vi "Manage logger file txt.vi"(0 "length":i32=1 min=1, 5 "Message to add":string, 11 "error in":errorcluster) -> (15 "error out":errorcluster)   [LabVIEW 2020]
panel:
  out "String":string
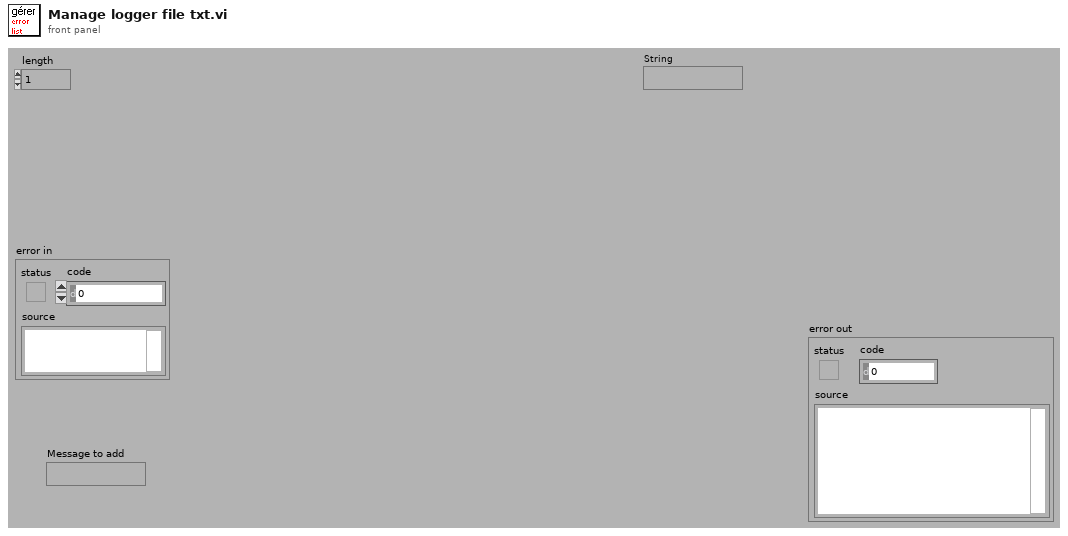
[diagram p1: front panel]
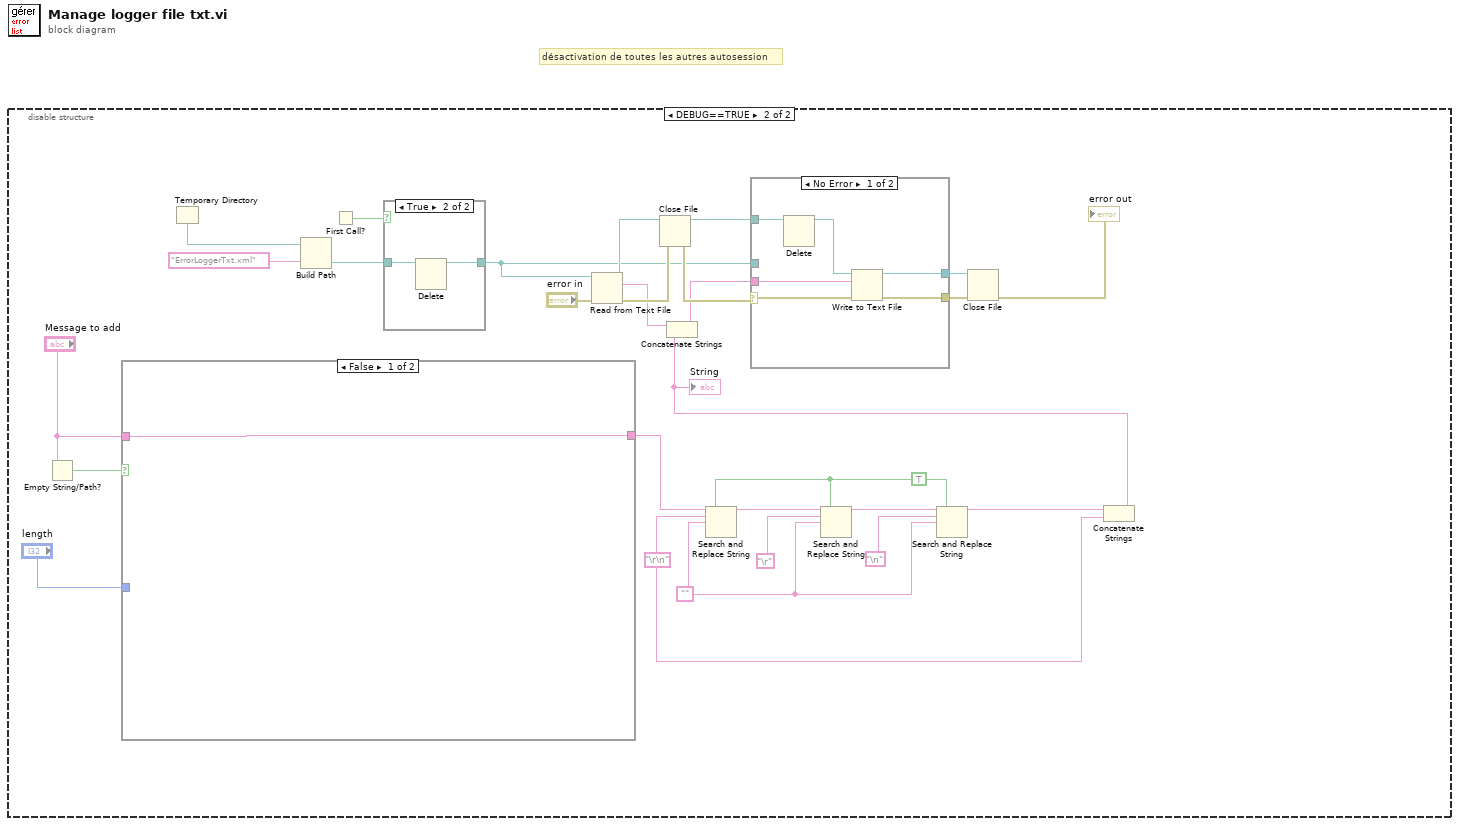
[diagram p0: block diagram]
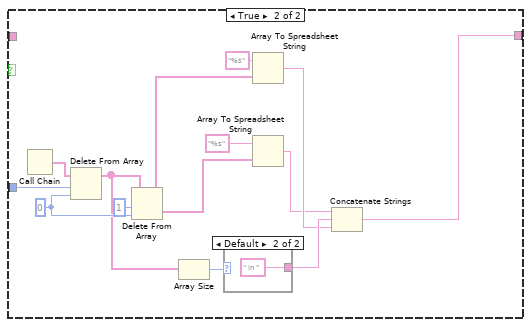
[diagram p3: hidden frame]
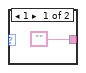
[diagram p4: hidden frame]
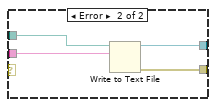
[diagram p6: hidden frame]
diagram:
  # "désactivation de toutes les autres autosession"
  n1 = disable-structure shown="DEBUG==TRUE" {
    frame condition #0 (active) {
    }
    frame condition #1 {
      w2 = "\r\n"
      w4 = ""
      w6 = TRUE ("replace all? (F)")
      n2 = Empty String/Path?(string/path="Message to add") -> (empty?=w13:bool)
      n3 = case shown="False" w13 {
        tunnel: [w29 w35] -> w1
        tunnel: "Message to add" -> [w29 _]
        tunnel: "length" -> [_ w34]
        frame False {
        }
        frame True {
          w39 = 0 ("Index")
          n4 = Call Chain() -> (call chain=w43:string[])
          n5 = Delete From Array(array=w43, length=w34, index=w39) -> (array with subset deleted=w36:string[])  [unwired: 1 out]
          n6 = Delete From Array(array=w36, length=1, index=w39) -> (deleted portion=w32:string[], array with subset deleted=w38:string[])
          n7 = Array Size(array=w36) -> (size(s)=w37:i32)
          n8 = case shown="Default" w37 {
            tunnel: ["" " in " ("Format String")] -> w42
            frame 1 {
            }
            frame Default {
            }
          }
          n9 = Array To Spreadsheet String(array=w38, 3:"%s" ("format string")) -> (spreadsheet string=w41:string)  [unwired: 1 in]
          n10 = Array To Spreadsheet String(array=w32, 3:"%s" ("format string")) -> (spreadsheet string=w31:string)  [unwired: 1 in]
          n11 = Concatenate Strings(w31, w42, w41) -> (w35:string)
        }
      }
      n12 = Temporary Directory() -> (w28:path)
      n13 = Build Path(base path=w28, name or relative path="ErrorLoggerTxt.xml") -> (appended path=w21:path)
      n14 = First Call?() -> (First Call?: T/F=w23:bool)
      n15 = case shown="True" w23 {
        tunnel: w21 -> [w46 w48]
        tunnel: [w46 w47] -> w22
        frame False {
        }
        frame True {
          n16 = Delete(path (use dialog)=w48) -> (deleted path=w47:path)  [unwired: 4 in, 2 out]
        }
      }
      n17 = Read from Text File(file (use dialog)=w22, error in="error in") -> (refnum out=w24:refnum<file>, text=w15:string, error out=w26:errorcluster)  [unwired: 2 in, 1 out]
      n18 = Close File(refnum=w24, error in=w26) -> (path=w25:path, error out=w27:errorcluster)
      n19 = Search and Replace String(replace all?=w6, input string=w1, search string=w2, replace string=w4) -> (result string=w5:string)  [unwired: 4 in, 3 out]
      n20 = Search and Replace String(replace all?=w6, input string=w5, search string="\r", replace string=w4) -> (result string=w8:string)  [unwired: 4 in, 3 out]
      n21 = Search and Replace String(replace all?=w6, input string=w8, search string="\n", replace string=w4) -> (result string=w3:string)  [unwired: 4 in, 3 out]
      n22 = Concatenate Strings(w3, w2) -> (w7:string)
      "String" <- w7
      n23 = Concatenate Strings(w15, w7) -> (w16:string)
      n24 = case shown="No Error" w27 {
        selector: w27 -> [w51 _]
        tunnel: w16 -> [w54 w58]
        tunnel: [w53 w57] -> w17
        tunnel: w22 -> [_ w56]
        tunnel: [w52 w55] -> w19
        tunnel: w25 -> [w50 _]
        frame No Error {
          n25 = Delete(path (use dialog)=w50) -> (deleted path=w49:path)  [unwired: 4 in, 2 out]
          n26 = Write to Text File(file (use dialog)=w49, text=w54, error in=w51) -> (refnum out=w53:refnum<file>, error out=w52:errorcluster)  [unwired: 1 in, 1 out]
        }
        frame Error {
          n27 = Write to Text File(file (use dialog)=w56, text=w58) -> (refnum out=w57:refnum<file>, error out=w55:errorcluster)  [unwired: 2 in, 1 out]
        }
      }
      n28 = Close File(refnum=w17, error in=w19) -> (error out=→"error out":errorcluster)  [unwired: 1 out]
    }
  }
